vi "Telemetry Event Loop.vi"(10 "Telemetry Notifier":refnum<notifier>) -> ()   [LabVIEW 2015]
uses:
  Telemetry Packet Type.ctl
  Thermocouple Data.ctl
  Connection Status Global Action.ctl
  System State Global Action.ctl
  System State.ctl
  Sequence Execution/Test Control Command.ctl
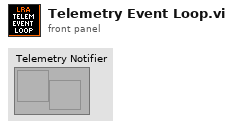
[diagram p1: front panel]
types:
  T1 = typedef "Connection Status Global Action.ctl" = enum16{"Get", "Set", "Initialize"}
  T2 = typedef "Test Control Command.ctl" = enum16{"Get Notifier", "Init", "Start", "Stop"}
  T3 = typedef "System State.ctl" = enum16{"Disabled", "E-Stop", "Standby", "Active"}
  T4 = typedef "System State Global Action.ctl" = enum16{"Get", "Set", "Initialize"}
  T5 = typedef "Telemetry Packet Type.ctl" = cluster{"Timestamp\n":u32, "Transducer Value":u16[], "Main Loop Rate":u32, "Solenoid State":bool[], "Output Enabled":bool, "Solenoids Powered":bool, "TC Data":T6[], "TD Rate":u32, "TD Execution Time":u32, "TC Rate":u32, "TC Execution Time":u32}
  T6 = typedef "Thermocouple Data.ctl" = cluster{"TC Temp":dbl, "Internal Temp":dbl, "Fault":bool, "Short to VCC":bool, "Short to GND":bool, "Open Circuit":bool}
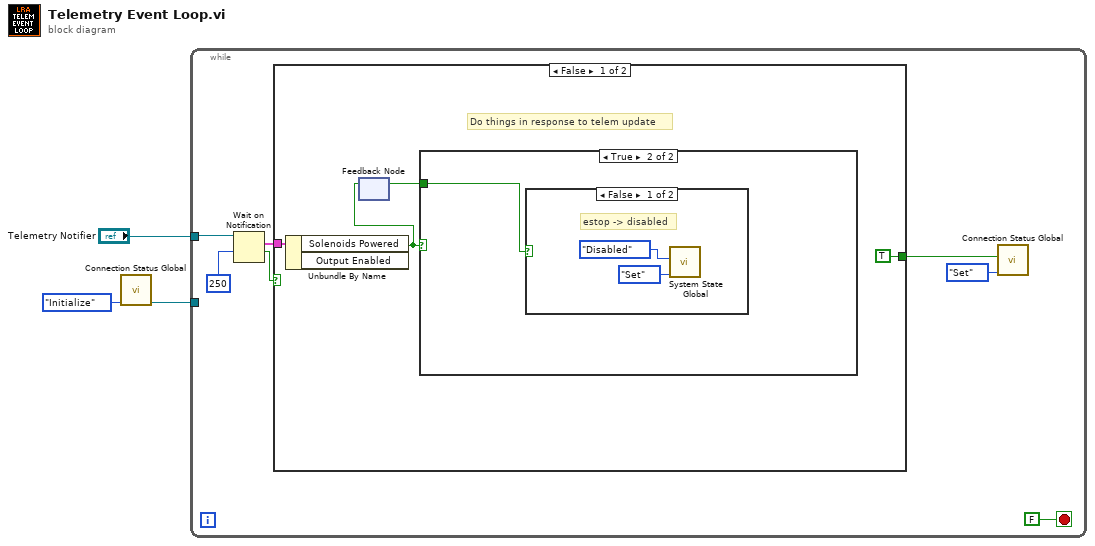
[diagram p0: block diagram]
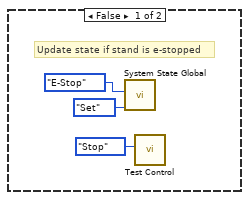
[diagram p2: hidden frame]
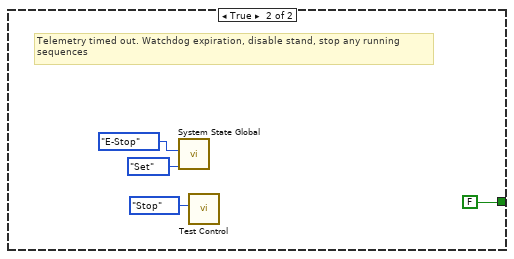
[diagram p4: hidden frame]
diagram:
  n1 = call "Connection Status Global.vi"("Operation"=Connection_Status_Global_Action."Initialize") -> ("Notifier"=w1:refnum<notifier>)  [unwired: 9 in, 1 out]
  n2 = while {
    tunnel: "Telemetry Notifier" -> [w9]
    tunnel: w1 -> [_]
    stop <- FALSE stop-if-true
    n3 = Wait on Notification(notifier=w9, timeout in ms (-1)=250) -> (notification=w8:T5, timed out?=w7:bool)  [unwired: 2 in, 2 out]
    n4 = case shown="False" w7 {
      tunnel: w8 -> [w14 _]
      tunnel: [TRUE FALSE] -> w4
      frame False {
        # "Do things in response to telem update"
        n5 = Unbundle By Name(w14) -> ("Solenoids Powered"=w12:bool)  [unwired: 1 out]
        n6 = feedback-in #1(w12) -> ()
        n7 = feedback #1() -> (w11:bool)  [unwired: 1 in]
        n8 = case shown="True" w12 {
          tunnel: w11 -> [_ w18]
          frame False {
            # "Update state if stand is e-stopped"
            n9 = call "System State Global.vi"("Action"=System_State_Global_Action."Set", "State In"=System_State."E-Stop") -> ()  [unwired: 8 in, 2 out]
            n10 = call "Test Control.vi"("Command"=Test_Control_Command."Stop") -> ()  [unwired: 10 in, 1 out]
          }
          frame True {
            n11 = case shown="False" w18 {
              frame False {
                # "estop -> disabled"
                n12 = call "System State Global.vi"("Action"=System_State_Global_Action."Set", "State In"=System_State."Disabled") -> ()  [unwired: 8 in, 2 out]
              }
              frame True {
              }
            }
          }
        }
      }
      frame True {
        # "Telemetry timed out. Watchdog expiration, disable stand, stop any running\nsequences"
        n13 = call "System State Global.vi"("Action"=System_State_Global_Action."Set", "State In"=System_State."E-Stop") -> ()  [unwired: 8 in, 2 out]
        n14 = call "Test Control.vi"("Command"=Test_Control_Command."Stop") -> ()  [unwired: 10 in, 1 out]
      }
    }
    n15 = call "Connection Status Global.vi"("Operation"=Connection_Status_Global_Action."Set", "Status In"=w4) -> ()  [unwired: 8 in, 2 out]
  }
